vi "mod_Rayleigh Fading (Jakes).vi"(0 "profile length (samples)":i32=1000, 5 "sampling frequency (Hz)":dbl=1.0 format="%.2f", 7 "doppler spread (Hz)":dbl=0.01 format="%.2p", 9 "seed in (0xFFFFFFFF)":i32=-1 format="%.0x", 11 "error in (no error)":errorcluster, 12 "fading variance":dbl=1.0 format="%.2f", 13 "reset? (T)":bool=TRUE) -> (4 "rayleigh fading profile":cdb[](array[numeric]) format="%.2f", 10 "next seed":i32=-1 format="%.0x", 15 "error out":errorcluster)   [LabVIEW 2020, in "niDMT.lvlib"]
doc: "The Rayleigh fading channel is generated based on Clarke and Gans Model using the Doppler filter with U-shaped power spectral density. \n \n\n Inputs:\n 1) Doppler spread (Hz) \n - range : double precision (default:20)\n - an example : a running vehicle with 65mph (104km/h), the carrier frequency of 900MHz\n The speed of the vehicle = 65*1.6*1000/3600 = 28.89m/s\n Doppler frequency = (900MHz)*(28.89m/s)/(300*10^6m/s) = 86.67 Hz\n 2) Fading variance : the variance of the fading channel output\n - range : double precision (default:2)\n 3) Input waveform : Input signal samples\n - some default values were set.\n (dt:0.00025, the number of samples:4000)\n 4) seed in (0xFFFFFFFF)\n 5) Error in\n\n Outputs:\n 1) Rayleigh fading profile : the complex fading channel output\n 2) Error out"
uses:
  <vilib>/addons/Modulation/niDMT.lvlib
  <vilib>/addons/Modulation/niAMT.lvlib
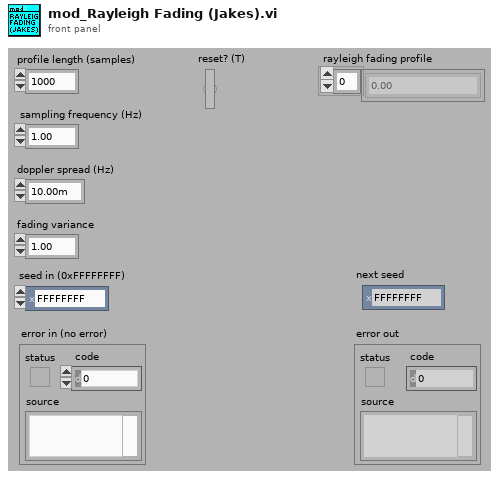
[diagram p1: front panel]
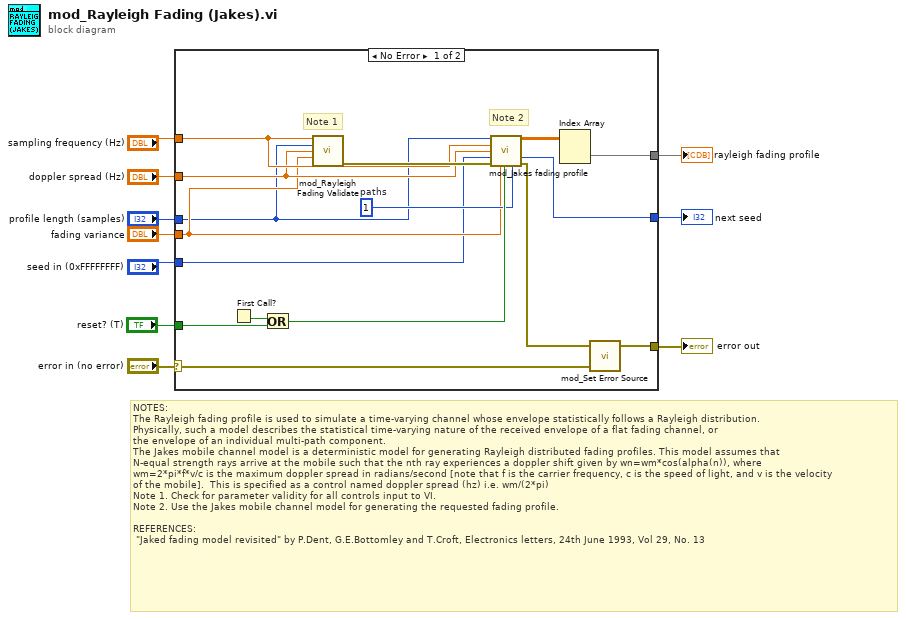
[diagram p0: block diagram]
diagram:
  # "NOTES:\nThe Rayleigh fading profile is used to simulate a time-varying channel whose envelope statistically follows a Rayleigh distribution. \nPhysically, such a model describes the statistical time-varying nature of the received envelope of a flat fading channel, or\nthe envelope of an individual multi-path component.\nThe Jakes mobile channel model is a deterministic model for generating Rayleigh distributed fading profiles. This model assumes that\nN-equal strength rays arrive at the mobile such that the nth ray experiences a doppler shift given by wn=wm*cos(alpha(n)), where \nwm=2*pi*f*v/c is the maximum doppler spread in radians/second [note that f is the carrier frequency, c is the speed of light, and v is the velocity \nof the mobile].  This is specified as a control named doppler spread (hz) i.e. wm/(2*pi)\nNote 1. Check for parameter validity for all controls input to VI.\nNote 2. Use the Jakes mobile channel model for generating the requested fading profile.\n\nREFERENCES:\n \"Jaked fading model revisited\" by P.Dent, G.E.Bottomley and T.Croft, Electronics letters, 24th June 1993, Vol 29, No. 13"
  n1 = case shown="No Error" "error in (no error)" {
    selector: "error in (no error)" -> [w25 w27]
    tunnel: [w26 w27] -> w10
    tunnel: [w20 _] -> w8
    tunnel: "sampling frequency (Hz)" -> [w17 _]
    tunnel: "doppler spread (Hz)" -> [w16 _]
    tunnel: "fading variance" -> [w15 _]
    tunnel: "profile length (samples)" -> [w14 _]
    tunnel: "seed in (0xFFFFFFFF)" -> [w13 _]
    tunnel: "reset? (T)" -> [w12 _]
    tunnel: [w11 _] -> w1
    frame No Error {
      w18 = u8 1  # paths
      # "Note 2"
      # "Note 1"
      n2 = First Call?() -> (First Call?: T/F=w24:bool)
      n3 = Or(x=w24, y=w12) -> (x .or. y?=w19:bool)
      n4 = call <vilib>:"mod_Rayleigh Fading Validate.vi"("sampling frequency"=w17, "profile length (samples)"=w14, "doppler spread (Hz)"=w16, "fading variance"=w15) -> ("error out"=w23:errorcluster)  [unwired: 11 out]
      n5 = call <vilib>:"mod_Jakes fading profile.vi"("profile length (samples)"=w14, "sampling frequency (hz)"=w17, "doppler spread (hz)"=w16, "seed in (0xFFFFFFFF)"=w13, "error in (no error)"=w23, "fading variance"=w15, "reset? (T)"=w19, "number of paths"=w18) -> ("fading profile"=w21:cdb[][], "next seed"=w11:i32, "error out"=w22:errorcluster)  [unwired: 5 out]
      n6 = Index Array(array=w21) -> (element=w20:cdb[])  [unwired: 2 in]
      n7 = call <vilib>:"mod_Set Error Source.vi"("initial error in (no error)"=w25, "final error in (no error)"=w22) -> ("error out"=w26:errorcluster)  [unwired: 1 in, 2 out]
    }
    frame Error {
    }
  }
  "error out" <- w10
  "rayleigh fading profile" <- w8
  "next seed" <- w1
